vi "WriteDataToDB.vi"(8 "通信协议名称":string, 9 "SN":refnum<vi>, 10 "产品型号":refnum<vi>, 11 "Slot":T1) -> (2 "ResultA":string, 3 "FSNA":string)   [LabVIEW 2013]
uses:
  SystemCode/SysControl/Slot.ctl
  GlobalValue.vi
  <vilib>/Utility/file.llb/Write To Spreadsheet File (string).vi
  <vilib>/Utility/file.llb/Read From Spreadsheet File (string).vi
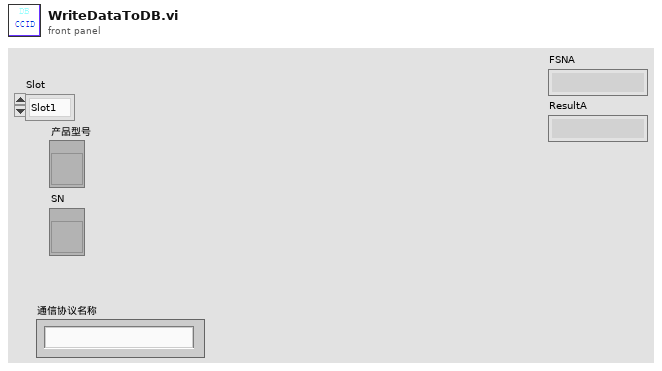
[diagram p1: front panel]
types:
  T1 = typedef "Slot.ctl" = enum16{"Slot1", "Slot2", "Slot3", "Slot4"}
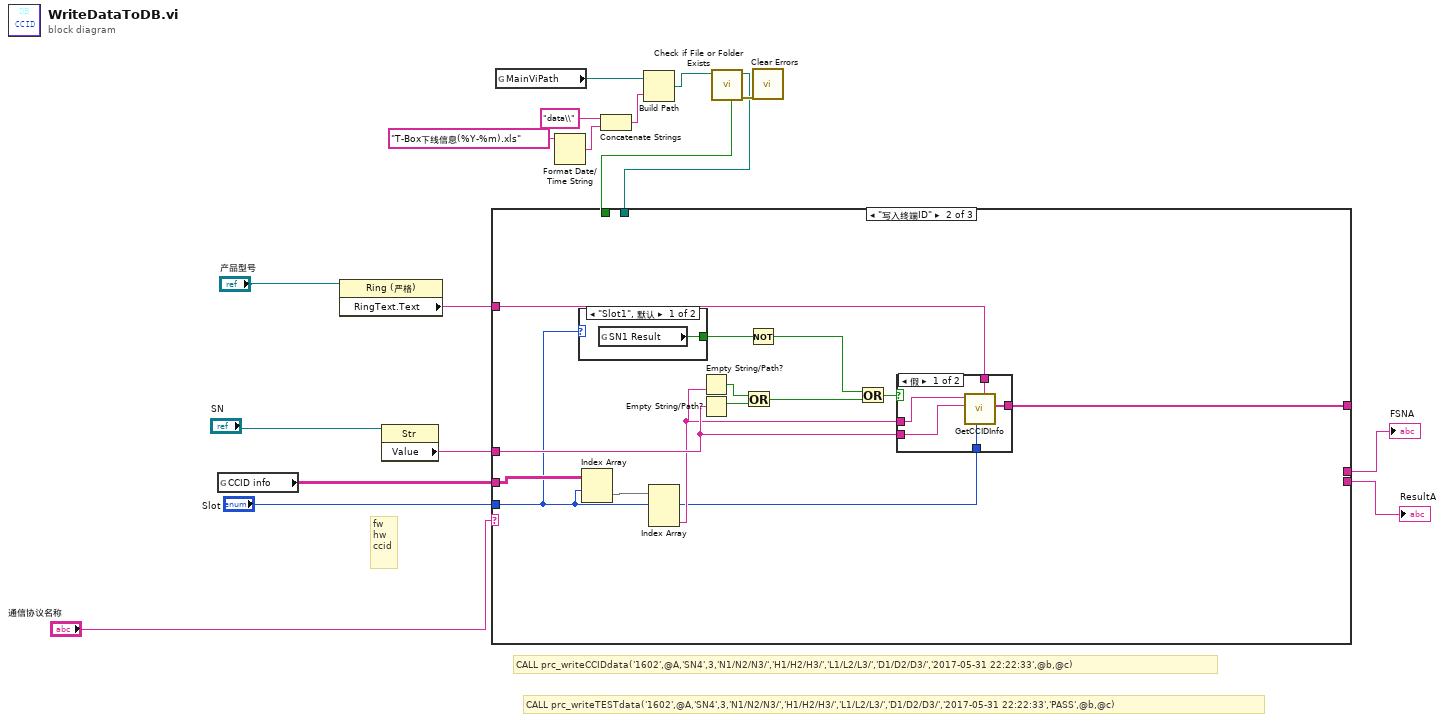
[diagram p0: block diagram]
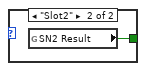
[diagram p3: hidden frame]
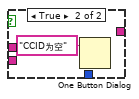
[diagram p4: hidden frame]
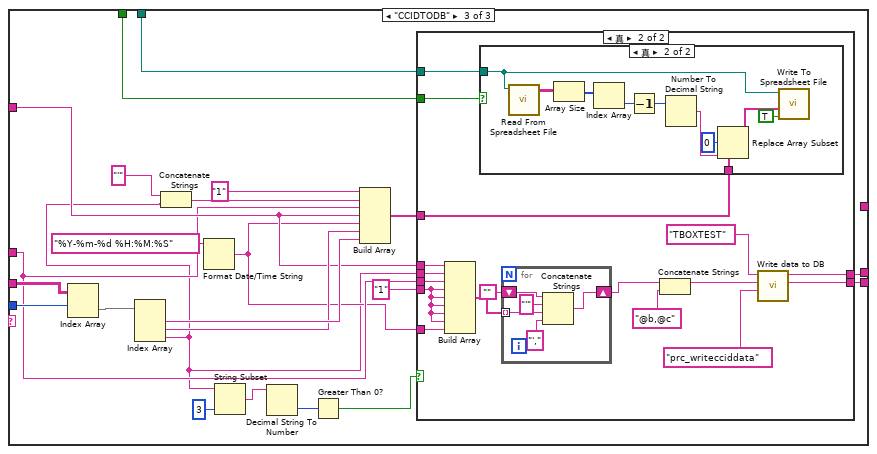
[diagram p5: hidden frame]
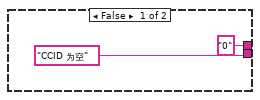
[diagram p6: hidden frame]
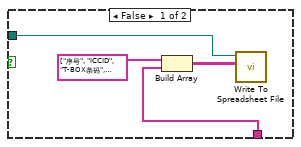
[diagram p7: hidden frame]
diagram:
  # "CALL prc_writeCCIDdata('1602',@A,'SN4',3,'N1/N2/N3/','H1/H2/H3/','L1/L2/L3/','D1/D2/D3/','2017-05-31 22:22:33',@b,@c)"
  # "CALL prc_writeTESTdata('1602',@A,'SN4',3,'N1/N2/N3/','H1/H2/H3/','L1/L2/L3/','D1/D2/D3/','2017-05-31 22:22:33','PASS',@b,@c)"
  # "fw\nhw\nccid"
  n1 = global read "GlobalValue.vi" "CCID info"() -> (w4:string[][])
  n2 = property class="Ring (严格)"(reference="产品型号") -> ("RingText.Text"=w18:string)  [unwired: 1 in, 2 out]
  n3 = property class="Str"(reference="SN") -> ("Value"=w17:string)  [unwired: 1 in, 2 out]
  n4 = global read "GlobalValue.vi" "MainViPath"() -> (w13:path)
  n5 = Format Date/Time String(time format string (%c)="T-Box下线信息(%Y-%m).xls" ("时间格式字符串(%c)")) -> (date/time string=w15:string)  [unwired: 2 in]
  n6 = Concatenate Strings("data\\" ("字符串"), w15) -> (w12:string)
  n7 = Build Path(base path=w13, name or relative path=w12) -> (appended path=w11:path)
  n8 = call <vilib>:"Check if File or Folder Exists.vi"("path"=w11) -> ("error out"=w10:errorcluster, "file or folder exists?"=w9:bool, "dup path"=w8:path)  [unwired: 8 in]
  n9 = case shown="\"写入终端ID\"" "通信协议名称" {
    tunnel: [_ w31 _] -> _
    tunnel: w18 -> [_ w24 w50]
    tunnel: w8 -> [_ _ w59]
    tunnel: w9 -> [_ _ w58]
    tunnel: w17 -> [_ w23 w49]
    tunnel: "Slot" -> [_ w19 w54]
    tunnel: w4 -> [_ w21 w55]
    tunnel: [_ _ w46] -> w2
    tunnel: [_ _ w45] -> w1
    frame "假", Default {
    }
    frame "写入终端ID" {
      n10 = case shown="\"Slot1\", 默认" w19 {
        tunnel: [w32 w33] -> w30
        frame "Slot1", Default {
          n11 = global read "GlobalValue.vi" "SN1 Result"() -> (w32:bool)
        }
        frame "Slot2" {
          n12 = global read "GlobalValue.vi" "SN2 Result"() -> (w33:bool)
        }
      }
      n13 = Index Array(array=w21, index (row)=w19) -> (element=w22:string[])  [unwired: 1 in]
      n14 = Index Array(array=w22) -> (element #3=w20:string)  [unwired: 3 in, 2 out]
      n15 = Empty String/Path?(string/path=w20) -> (empty?=w29:bool)
      n16 = Empty String/Path?(string/path=w23) -> (empty?=w28:bool)
      n17 = Or(x=w29, y=w28) -> (x .or. y?=w26:bool)
      n18 = Not(x=w30) -> (.not. x?=w27:bool)
      n19 = Or(x=w27, y=w26) -> (x .or. y?=w25:bool)
      n20 = case shown="假" w25 {
        tunnel: [w38 _] -> w31
        tunnel: w20 -> [w37 _]
        tunnel: w23 -> [w36 _]
        tunnel: w24 -> [w35 _]
        tunnel: w19 -> [w34 _]
        frame False {
          n21 = call "GetCCIDInfo.vi"("table name"=w35, "Slot"=w34, "SerNO"=w36, "CCID"=w37) -> ("CCID信息"=w38:string[])  [unwired: 7 in]
        }
        frame True {
          n22 = One Button Dialog(message="CCID为空" ("消息")) -> ()  [unwired: 1 in, 1 out]
        }
      }
    }
    frame "CCIDTODB" {
      n23 = Index Array(array=w55, index (row)=w54) -> (element=w53:string[])  [unwired: 1 in]
      n24 = Index Array(array=w53) -> (element #1=w52:string, element #2=w51:string, element #3=w44:string)  [unwired: 3 in]
      n25 = Concatenate Strings("'", w44) -> (w56:string)
      n26 = Format Date/Time String(time format string (%c)="%Y-%m-%d %H:%M:%S" ("时间格式字符串(%c)")) -> (date/time string=w48:string)  [unwired: 2 in]
      n27 = String Subset(string=w44, length (rest)=3 ("长度（剩余）")) -> (substring=w42:string)  [unwired: 1 in]
      n28 = Decimal String To Number(string=w42) -> (number=w41:i32)  [unwired: 2 in, 1 out]
      n29 = Greater Than 0?(x=w41) -> (x > 0?=w40:bool)
      n30 = Build Array("1", w56, w49, w50, w48, w51, w52) -> (w60:string[])
      n31 = case shown="真" w40 {
        tunnel: w60 -> [_ w81]
        tunnel: w59 -> [_ w80]
        tunnel: w58 -> [_ w79]
        tunnel: w50 -> [_ w76]
        tunnel: w49 -> [_ w75]
        tunnel: w48 -> [_ w74]
        tunnel: "1" ("元素") -> [_ w73]
        tunnel: ["0" ("FSNA") w67] -> w46
        tunnel: ["CCID 为空" ("ResultA") w66] -> w45
        tunnel: w44 -> [_ w65]
        frame False {
        }
        frame True {
          n32 = Build Array(w76, w65, w75, w73, w73, w73, w73, w73, w74) -> (w72:string[])
          n33 = case shown="真" w79 {
            tunnel: w80 -> [w90 w91]
            tunnel: w81 -> [w89 w95]
            frame False {
              n34 = Build Array(string[] ["序号", "ICCID", "T-BOX条码", "设备型号", "生产日期", "硬件版本", "软件版本"], w89) -> (w88:string[][])
              n35 = call-poly <vilib>:"Write To Spreadsheet File.vi"("2D data"=w88, "file path (dialog if empty)"=w90) -> ()  [unwired: 6 in, 1 out]
            }
            frame True {
              n36 = call-poly <vilib>:"Read From Spreadsheet File.vi"("file path (dialog if empty)"=w91) -> ("all rows"=w100:string[][])  [unwired: 6 in, 4 out]
              n37 = Array Size(array=w100) -> (size(s)=w99:i32[])
              n38 = Index Array(array=w99) -> (element=w98:i32)  [unwired: 1 in]
              n39 = Decrement(x=w98) -> (x-1=w97:i32)
              n40 = Number To Decimal String(number=w97) -> (decimal integer string=w93:string)  [unwired: 1 in]
              n41 = Replace Array Subset(array=w95, new element=w93, index=0 ("索引")) -> (w92:string[])
              n42 = call-poly <vilib>:"Write To Spreadsheet File.vi"("append to file? (new file:F)"=TRUE, "1D data"=w92, "file path (dialog if empty)"=w91) -> ()  [unwired: 5 in, 1 out]
            }
          }
          n43 = for {
            tunnel: w72 -> [w83] mode=indexing
            shift-right: [w85] -> w70
            shift-left: "" -> [w84]
            n44 = Concatenate Strings(w84, "'" ("字符串"), w83, "',") -> (w85:string)
          }
          n45 = Concatenate Strings(w70, "@b,@c" ("元素")) -> (w68:string)
          n46 = call "Write data to DB.vi"("Procedure name"="prc_writecciddata", "all string"=w68, "DSN name"="TBOXTEST") -> ("ResultA"=w66:string, "FSNA"=w67:string)  [unwired: 6 in, 1 out]
        }
      }
    }
  }
  "FSNA" <- w2
  "ResultA" <- w1
  n47 = call <vilib>:"Clear Errors.vi"("error in (no error)"=w10) -> ()  [unwired: 6 in, 1 out]
